vi "OculusRift INTERFACE VI_UDP_test.vi"() -> ()   [LabVIEW 2014]
uses:
  <vilib>/Platform/TimedLoop/XDataNode/timing_clust.ctl
  <vilib>/Platform/TimedLoop/XDataNode/nitl_modes.ctl
  <vilib>/Platform/TimedLoop/XDataNode/wakeup.ctl
  <vilib>/Platform/TimedLoop/XDataNode/XDataNode.xnode
  <vilib>/Platform/TimedLoop/XDataNode/XDNodeRunTimeDep.lvlib
panel:
  in  "Remote UDP port 2":u16=6340
  in  "Local UDP port":u16=6340
  in  "error in (no error) 3":errorcluster
  in  "Ip":string="localhost"
  in  "LOOP CS":i64=200
  in  "LOOP OR":i64
  out "error out":errorcluster
  out "data out":string
  in  "error in (no error)":errorcluster
  in  "OR Port":u16=52717
  in  "Oculus Rift Adress":string="localhost"
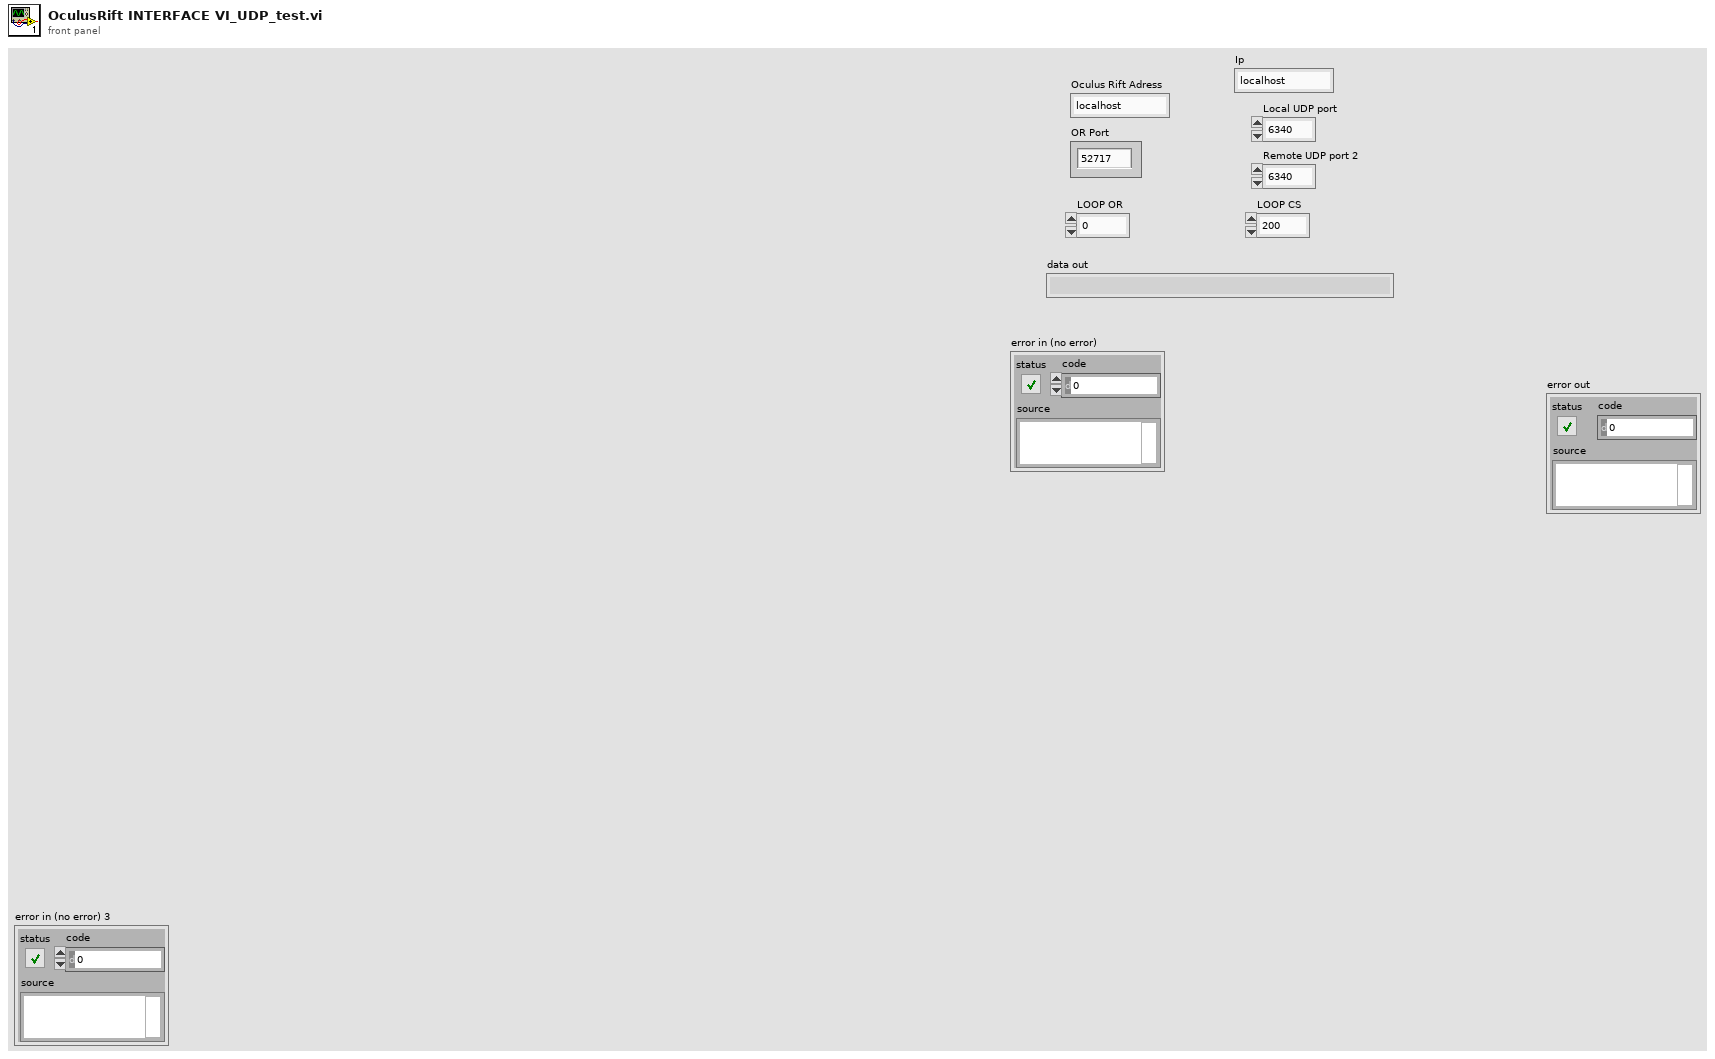
[diagram p1: front panel]
types:
  T1 = typedef "XDNodeRunTimeDep.lvlib/timing_clust.ctl" = cluster{"Expected End [f-1]":u64, "Actual End [f-1]":u64, "Finished Late? [f-1]":bool, "Expected End [i-1]":u64, "Actual End [i-1]":u64, "Finished Late? [i-1]":bool, "Expected Start [i]":u64, "Actual Start [i]":u64, "Expected Start [f]":u64, "Actual Start [f]":u64, "Source Name":string, "Structure Name":string, "Period":i64, "Deadline":i64, "Offset":i64, "Start":i64, "Priority":i32, "Timeout":i32, "Mode":T2, "Wakeup Reason":T3, "Error":errorcluster, "Source Type":string, "Secondary Source Type":string, "Global End Time":u64, "Global Start Time":u64, "Frame Duration":u64, "Iteration Duration":u64, "Assigned CPU":i32, "I/O Scan Engine Mode":u32}
  T2 = typedef "XDNodeRunTimeDep.lvlib/nitl_modes.ctl" = enum32{"No Change", "Process missed periods, maintain original phase", "Discard missed periods, maintain original phase", "Process missed periods, ignore original phase", "Discard missed periods, ignore original phase"}
  T3 = typedef "XDNodeRunTimeDep.lvlib/wakeup.ctl" = enum32{"Normal", "Aborted", "Asynchronous wakeup", "Timing source error", "Timed loop error", "Timeout"}
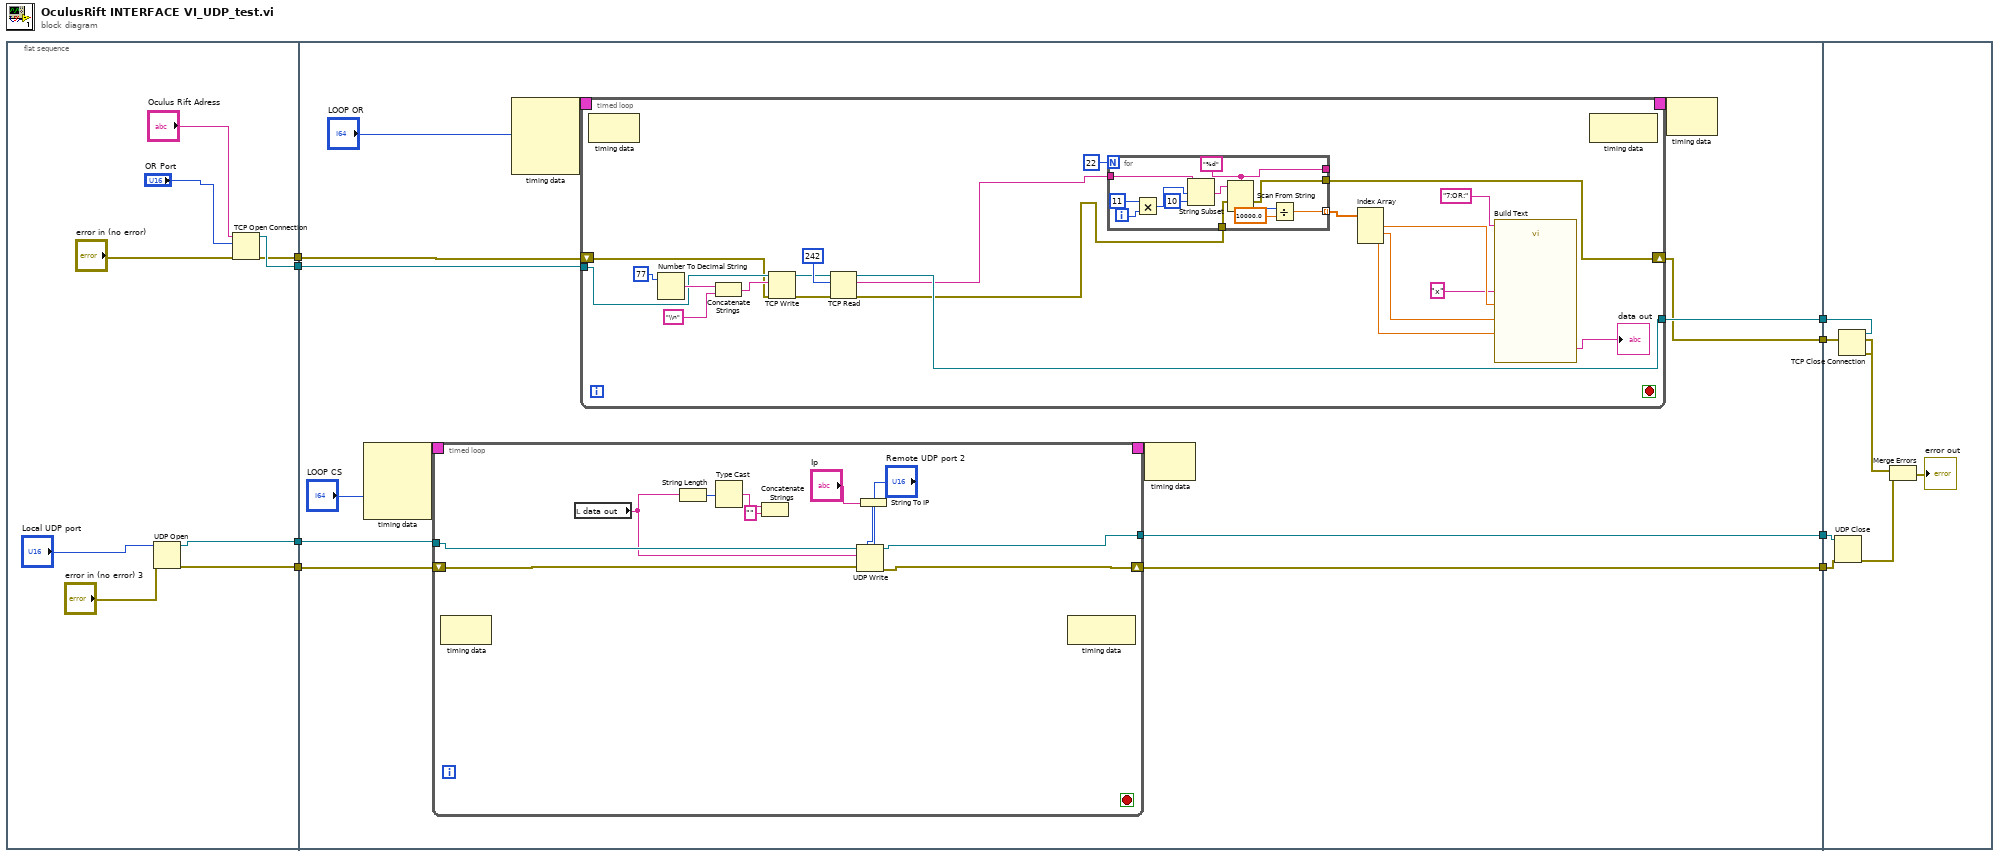
[diagram p0: block diagram]
diagram:
  n1 = flat-sequence {
    tunnel: [w17] -> w8
    tunnel: [w16] -> w7
    tunnel: [w10] -> w2
    tunnel: [w9] -> w1
    tunnel: w8 -> [w29]
    tunnel: w7 -> [w28]
    tunnel: [w27] -> w6
    tunnel: [w26] -> w5
    tunnel: [w25] -> w4
    tunnel: [w24] -> w3
    tunnel: w2 -> [w19]
    tunnel: w1 -> [w18]
    tunnel: w6 -> [w88]
    tunnel: w5 -> [w89]
    tunnel: w4 -> [w94]
    tunnel: w3 -> [w93]
    frame #0 {
      n2 = UDP Open(8:"error in (no error) 3", 11:"Local UDP port") -> (port=w10:refnum<k16>, 0:w9:errorcluster)  [unwired: 3 in, 1 out]
      n3 = TCP Open Connection(address="Oculus Rift Adress", remote port or service name="OR Port", error in (no error)="error in (no error)") -> (connection ID=w17:refnum<k5>, error out=w16:errorcluster)  [unwired: 2 in]
    }
    frame #1 {
      n4 = node-c288("LOOP CS") -> (w31:T1)  [unwired: 3 in]
      n5 = timed-loop {
        timing: w31 -> [_]
        timing-out: [_] -> w30
        shift-right: [w78] -> w26
        shift-left: w18 -> [w77]
        tunnel: [w79] -> w27
        tunnel: w19 -> [w75]
        stop <- _ stop-if-true
        n6 = node-c288() -> ()  [unwired: 1 in, 1 out]
        n7 = local read "data out"() -> (w72:string)
        n8 = String Length(string=w72) -> (length=w81:i32)
        n9 = Type Cast(x=w81) -> (*(type *) &x=w80:string)  [unwired: 1 in]
        n10 = Concatenate Strings(w80, "" ("string")) -> ()  [unwired: 1 out]
        n11 = String To IP(1:"Ip") -> (0:w76:u32)
        n12 = UDP Write(address=w76, port or service name="Remote UDP port 2", connection ID=w75, data in=w72, 8:w77) -> (error out=w78:errorcluster, 3:w79:refnum<k16>)  [unwired: 1 in]
        n13 = node-c288() -> ()  [unwired: 1 in, 1 out]
      }
      n14 = node-c288("LOOP OR") -> (w22:T1)  [unwired: 3 in]
      n15 = timed-loop {
        timing: w22 -> [_]
        timing-out: [_] -> w21
        tunnel: w29 -> [w45]
        shift-right: [w33] -> w24
        shift-left: w28 -> [w44]
        tunnel: [w43] -> w25
        stop <- _ stop-if-true
        n16 = node-c288() -> ()  [unwired: 1 in, 1 out]
        n17 = Number To Decimal String(number=77) -> (decimal integer string=w48:string)  [unwired: 1 in]
        n18 = Concatenate Strings(w48, "\\n" ("string")) -> (w46:string)
        n19 = TCP Write(connection ID=w45, data in=w46, error in (no error)=w44) -> (connection ID out=w51:refnum<k5>, error out=w50:errorcluster)  [unwired: 1 in, 1 out]
        n20 = TCP Read(connection ID=w51, bytes to read=242, error in (no error)=w50) -> (connection ID out=w43:refnum<k5>, data out=w36:string, error out=w34:errorcluster)  [unwired: 2 in]
        n21 = for {
          N: 22 -> [_]
          tunnel: w36 -> [w64]
          tunnel: [w57] -> w40 mode=indexing
          tunnel: w34 -> [w55]
          tunnel: [w54] -> w33
          tunnel: [w53] -> _
          i -> [w62]
          w53 = "%d" ("format string")
          n22 = Multiply(x=11, y=w62) -> (x*y=w60:i32)
          n23 = String Subset(string=w64, offset (0)=w60, length (rest)=10 ("length (rest)")) -> (substring=w59:string)
          n24 = Scan From String(format string=w53, input string=w59, error in=w55) -> (error out=w54:errorcluster, output 1=w56:i32)  [unwired: 2 in, 2 out]
          n25 = Divide(x=w56, y=10000.0) -> (x/y=w57:dbl)
        }
        n26 = Index Array(array=w40) -> (element #1=w39:dbl, element #2=w38:dbl, element #3=w37:dbl)  [unwired: 3 in]
        n27 = call "Build Text"("Beginning Text"="7:OR:", "val3"=w37, "ORStatus"="x", "val1"=w39, "val2"=w38) -> ("Result"=→"data out":string)  [unwired: 9 in, 1 out]
        n28 = node-c288() -> ()  [unwired: 1 in, 1 out]
      }
      n29 = node-c288(w30) -> ()  [unwired: 1 out]
      n30 = node-c288(w21) -> ()  [unwired: 1 out]
    }
    frame #2 {
      n31 = UDP Close(connection ID=w88, 8:w89) -> (error out=w90:errorcluster)  [unwired: 1 out]
      n32 = TCP Close Connection(connection ID=w94, error in (no error)=w93) -> (error out=w92:errorcluster)  [unwired: 1 in, 1 out]
      n33 = Merge Errors(w92, w90) -> (→"error out":errorcluster)
    }
  }
